vi "Measurement Logic.vi"(8 "error in":errorcluster, 10 "Measurement Context":refnum<class "MeasurementContext.lvclass">, 11 "Measurement Configuration":T2) -> (0 "error out":errorcluster, 2 "Measurement Context out":refnum<class "MeasurementContext.lvclass">, 3 "Measurement Results":T1)   [LabVIEW 2020, in "MeasurementLink Measurement Template.lvlib"]
uses:
  MeasurementLink Measurement Template.lvlib
  Measurement Configuration.ctl
  Measurement Results.ctl
  MeasurementLink Measurement Server/Classes/MeasurementContext/MeasurementContext.lvclass
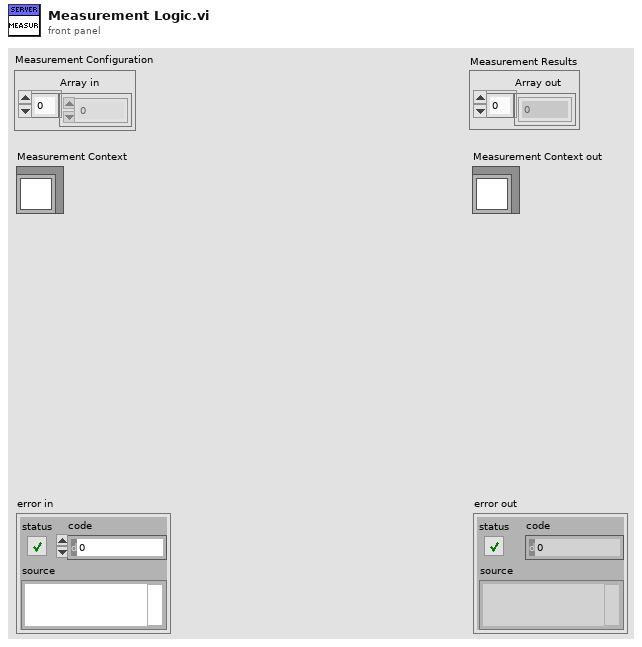
[diagram p1: front panel]
types:
  T1 = typedef "MeasurementLink Measurement Template.lvlib/Measurement Results.ctl" = cluster{"Array out":dbl[]}
  T2 = typedef "MeasurementLink Measurement Template.lvlib/Measurement Configuration.ctl" = cluster{"Array in":dbl[]}
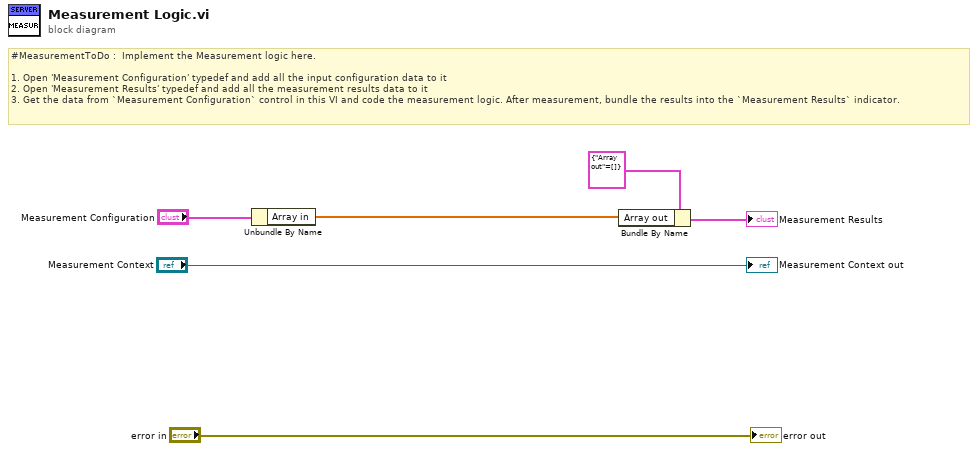
[diagram p0: block diagram]
diagram:
  # "#MeasurementToDo :  Implement the Measurement logic here.\n\n1. Open 'Measurement Configuration' typedef and add all the input configuration data to it\n2. Open 'Measurement Results' typedef and add all the measurement results data to it\n3. Get the data from `Measurement Configuration` control in this VI and code the measurement logic. After measurement, bundle the results into the `Measurement Results` indicator."
  n1 = Unbundle By Name("Measurement Configuration") -> ("Array in"=w3:dbl[])
  n2 = Bundle By Name(cluster=T1 {"Array out"=[]} ("Measurement Results"), "Array out"=w3) -> (→"Measurement Results":T1)
  "error out" <- "error in"
  "Measurement Context out" <- "Measurement Context"
